vi "Load.vi"(8 "error in":errorcluster, 11 "DNL_Font":refnum<vi>) -> (0 "error out":errorcluster, 3 "INI Data":T1 {"Body Text"."Body Text Spec"."Alignment" items=["left", "center", "right"]; "Text"."Alignment" items=["left", "center", "right"]})   [LabVIEW 2021]
uses:
  Controls/INI.ctl
  vi.lib/LabVIEW Icon API/lv_icon/Controls/Font.ctl
  vi.lib/LabVIEW Icon API/lv_icon/Controls/Alignment.ctl
  Controls/Font Size.ctl
  vi.lib/LabVIEW Icon API/lv_icon/Controls/BodyText.ctl
  vi.lib/LabVIEW Icon API/lv_icon/Controls/IEColor.ctl
  Controls/Tools.ctl
  Controls/Pen.ctl
  Controls/Line.ctl
  Controls/Dropper.ctl
  Controls/Fill.ctl
  Controls/IERect.ctl
  Controls/FRect.ctl
  Controls/Circle.ctl
  Controls/FCircle.ctl
  Controls/Rubber.ctl
  Controls/Text.ctl
  Controls/Selection.ctl
  Controls/Move.ctl
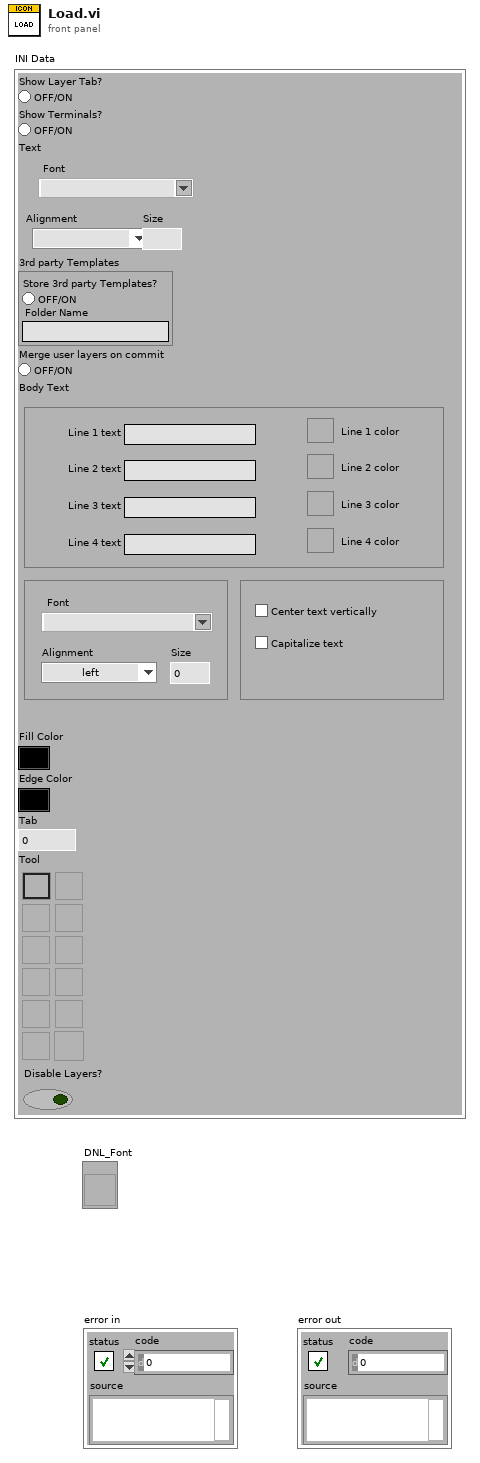
[diagram p1: front panel]
types:
  T1 = typedef "INI.ctl" = cluster{"Show Layer Tab?":bool, "Show Terminals?":bool, "Text":cluster{"Font":T2, "Alignment":T3, "Size":T4}, "3rd party Templates":cluster{"Store 3rd party Templates?":bool, "Folder Name":string}, "Merge user layers on commit":bool, "Body Text":T5, "Fill Color":T6, "Edge Color":T6, "Tab":u16, "Tool":T7, "Disable Layers?":bool}
  T2 = typedef "Font.ctl" = string
  T3 = typedef "Alignment.ctl" = u16
  T4 = typedef "Font Size.ctl" = u8
  T5 = typedef "BodyText.ctl" = cluster{"Line 1 text":string, "Line 2 text":string, "Line 3 text":string, "Line 4 text":string, "Line 1 color":u32, "Line 2 color":u32, "Line 3 color":u32, "Line 4 color":u32, "Body Text Spec":cluster{"Font":T2, "Alignment":T3, "Size":u8}, "Center text vertically":bool, "Capitalize Text":bool}
  T6 = typedef "IEColor.ctl" = u32
  T7 = typedef "Tools.ctl" = enum32{"Pencil", "Line", "Dropper", "Fill", "Rectangle", "Filled Rectangle", "Ellipse", "Filled Ellipse", "Eraser", "Text", "Select", "Move"}
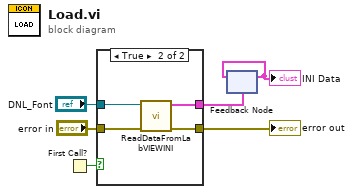
[diagram p0: block diagram]
diagram:
  n1 = First Call?() -> (First Call?: T/F=w6:bool)
  n2 = case shown="True" w6 {
    tunnel: [w7 w10] -> w4
    tunnel: [_ w9] -> w3
    tunnel: "error in" -> [w7 w11]
    tunnel: "DNL_Font" -> [_ w8]
    frame False {
    }
    frame True {
      n3 = call "ReadDataFromLabVIEWINI.vi"("error in (no error)"=w11, "DNL_Font"=w8) -> ("error out"=w10:errorcluster, "INI Data"=w9:T1)  [unwired: 8 out]
    }
  }
  "error out" <- w4
  n4 = feedback #1(w3) -> (w2:T1)
  "INI Data" <- w2
  n5 = feedback-in #1(w2) -> ()
